vi "SetTriggerImpedance.vi"(2 "error in (no error)":errorcluster, 3 "Trigger IN Impedance":u8(ring) items=["50 Ohm", "1K Ohm"], 4 "VISA resource name":refnum<visa-resource-name>) -> (0 "error out":errorcluster, 1 "VISA resource name out":refnum<visa-resource-name>)   [LabVIEW 2020, in "Active Technologies AWG3000.lvlib"]
uses:
  Active Technologies AWG3000.lvlib
panel:
  out "VISA STRING":string
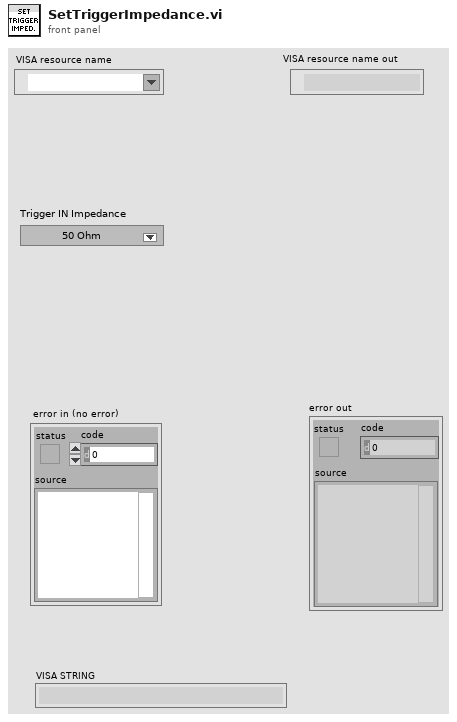
[diagram p1: front panel]
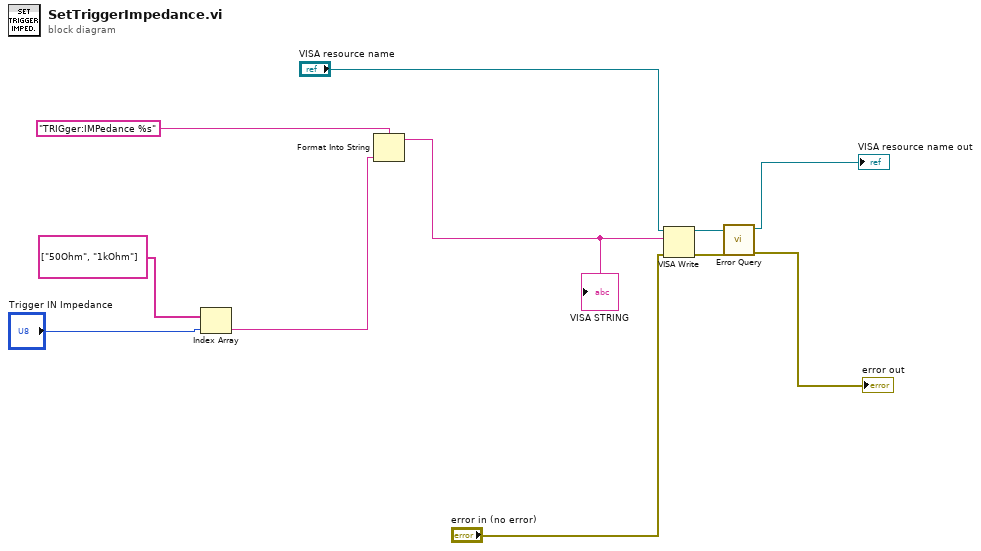
[diagram p0: block diagram]
diagram:
  n1 = Index Array(array=string[] ["50Ohm", "1kOhm"], index="Trigger IN Impedance") -> (element=w2:string)
  n2 = Format Into String(format string="TRIGger:IMPedance %s" ("write buffer"), w2) -> (resulting string=w1:string)  [unwired: 2 in, 1 out]
  "VISA STRING" <- w1
  n3 = VISA Write(VISA resource name="VISA resource name", write buffer=w1, error in (no error)="error in (no error)") -> (VISA resource name out=w9:refnum<visa-resource-name>, error out=w8:errorcluster)  [unwired: 1 out]
  n4 = call "Error Query.vi"("error in (no error)"=w8, "VISA resource name"=w9) -> ("error out"=→"error out":errorcluster, "VISA resource name out"=→"VISA resource name out":refnum<visa-resource-name>)  [unwired: 6 in, 2 out]
